vi "Signals+Noise.vi"() -> ()   [LabVIEW 2020]
uses:
  <vilib>/Analysis/2dsp.llb/Real FFT.vi
  <vilib>/Analysis/NI_AALBase.lvlib
  <vilib>/Analysis/NI_AALPro.lvlib
panel:
  out "FFT":dbl[](graph)
  out "Graph":dbl[](graph)
  in  "reset signal":bool
  in  "noise (rms)":dbl=0.2 format="%.2f"
  in  "offset":dbl format="%.2p"
  in  "seed":i32=-1
  out "error":i32
  in  "Fs":dbl=1000.0 format="%.2p"
  in  "samples":i32=128
  in  "tones":T1(array[cluster])=[{"frequency"=10.0, "amplitude"=1.0, "phase"=0.0}, {"frequency"=20.0, "amplitude"=0.1, "phase"=0.0}, {"frequency"=60.0, "amplitude"=1.0, "phase"=0.0}] {"phase" format="%0.2f"; "amplitude" format="%0.2p"; "frequency" format="%0.2p"}
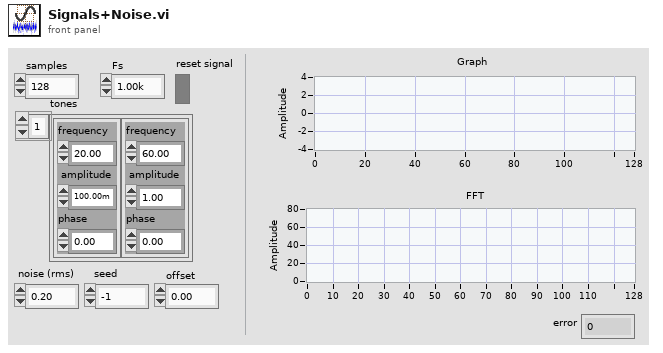
[diagram p1: front panel]
types:
  T1 = cluster{"frequency":dbl, "amplitude":dbl, "phase":dbl}[]
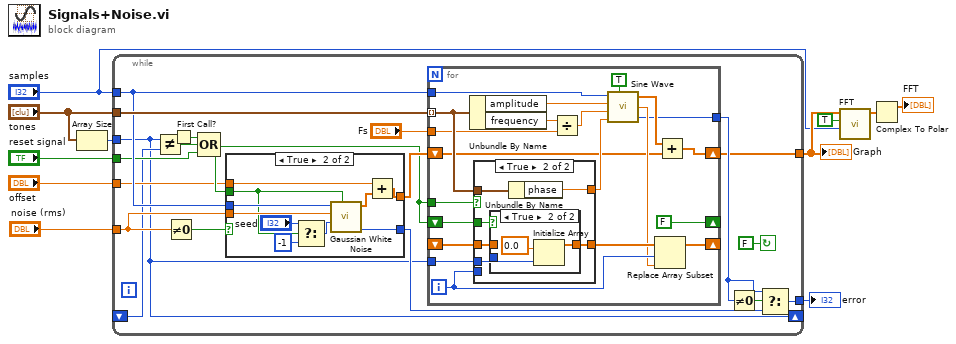
[diagram p0: block diagram]
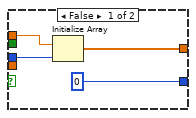
[diagram p2: hidden frame]
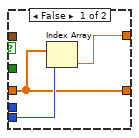
[diagram p3: hidden frame]
diagram:
  n1 = Array Size(array="tones") -> (size(s)=w9:i32)
  n2 = while {
    shift-right: [w12] -> _
    shift-left: _ -> [w13]
    tunnel: "tones" -> [w22]
    tunnel: "samples" -> [w21]
    tunnel: "reset signal" -> [w20]
    tunnel: w9 -> [w12]
    tunnel: "offset" -> [w17]
    tunnel: "noise (rms)" -> [w16]
    tunnel: [w15] -> w5
    tunnel: [w14] -> w6
    stop <- FALSE continue-if-true
    n3 = Not Equal?(x=w12, y=w13) -> (x != y?=w19:bool)
    n4 = Not Equal To 0?(x=w16) -> (x != 0?=w30:bool)
    n5 = First Call?() -> (First Call?: T/F=w18:bool)
    n6 = Compound Arithmetic op=OR(w18, w19, w20) -> (w28:bool)
    n7 = case shown="True" w30 {
      tunnel: w16 -> [_ w44]
      tunnel: w17 -> [w32 w42]
      tunnel: w21 -> [w34 w43]
      tunnel: [w33 w41] -> w29
      tunnel: [0 ("error") w39] -> w25
      tunnel: w28 -> [_ w35]
      frame False {
        n8 = Initialize Array(w32, w34) -> (w33:dbl[])
      }
      frame True {
        n9 = Select(t="seed", s=w35, f=-1) -> (s? t:f=w36:i32)
        n10 = call <vilib>:"Gaussian White Noise.vi"("initialize?"=w35, "seed"=w36, "standard deviation"=w44, "samples"=w43) -> ("error"=w39:i32, "Gaussian noise pattern"=w40:dbl[])  [unwired: 6 in]
        n11 = Add(x=w42, y=w40) -> (x+y=w41:dbl[])
      }
    }
    n12 = for {
      tunnel: w22 -> [w64] mode=indexing
      shift-right: [w65] -> w15
      shift-left: w29 -> [w51]
      shift-right: [w60] -> _
      shift-left: _ -> [w62]
      tunnel: w21 -> [w49]
      tunnel: [w50] -> w26
      tunnel: w28 -> [w52]
      shift-right: [FALSE] -> _
      shift-left: w28 -> [w48]
      tunnel: "Fs" -> [w46]
      tunnel: w12 -> [w45]
      i -> [w61]
      n13 = Unbundle By Name(w64) -> ("amplitude"=w55:dbl, "frequency"=w57:dbl)
      n14 = case shown="True" w52 {
        tunnel: w64 -> [_ w74]
        tunnel: [w67 w73] -> w59
        tunnel: w45 -> [_ w71]
        tunnel: [w66 w72] -> w63
        tunnel: w62 -> [w66 w69]
        tunnel: w61 -> [w68 _]
        tunnel: w48 -> [_ w70]
        frame False {
          n15 = Index Array(array=w66, index=w68) -> (element=w67:dbl)
        }
        frame True {
          n16 = case shown="True" w70 {
            tunnel: [w75 w77] -> w72
            tunnel: w71 -> [_ w76]
            tunnel: w69 -> [w75 _]
            frame False {
            }
            frame True {
              n17 = Initialize Array(0.0 ("element"), w76) -> (w77:dbl[])
            }
          }
          n18 = Unbundle By Name(w74) -> ("phase"=w73:dbl)
        }
      }
      n19 = Divide(x=w57, y=w46) -> (x/y=w56:dbl)
      n20 = call <vilib>:"Sine Wave.vi"("samples"=w49, "amplitude"=w55, "frequency"=w56, "phase in"=w59, "reset phase"=TRUE ("reset signal")) -> ("sine wave"=w54:dbl[], "phase out"=w58:dbl, "error"=w50:i32)
      n21 = Replace Array Subset(array=w63, new element=w58, index=w61) -> (w60:dbl[])
      n22 = Add(x=w54, y=w51) -> (x+y=w65:dbl[])
    }
    n23 = Not Equal To 0?(x=w26) -> (x != 0?=w27:bool)
    n24 = Select(t=w26, s=w27, f=w25) -> (s? t:f=w14:i32)
  }
  "error" <- w6
  "Graph" <- w5
  n25 = call-poly <vilib>:"FFT.vi"("FFT size"="samples", "shift?"=TRUE, "X"=w5) -> ("FFT {X}"=w2:cdb[])  [unwired: 7 in, 1 out]
  n26 = Complex To Polar(r * e^(i*theta)=w2) -> (r=→"FFT":dbl[])  [unwired: 1 out]
